vi "Build.vi"(6 "Assembly Type":string, 8 "Position":i32, 9 "XYZTheta":dbl[](array[numeric]), 10 "Pattern Coordinates":dbl[][](array[numeric]), 11 "Dispense in":refnum<class "Dispense.lvclass">) -> (3 "Dispense out":refnum<class "Dispense.lvclass">)   [LabVIEW 2021, in "Dispense.lvclass"]
uses:
  Dispense.lvclass
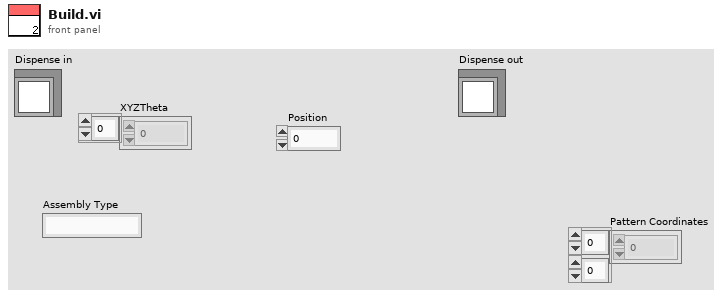
[diagram p1: front panel]
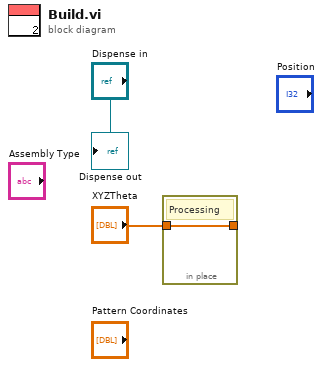
[diagram p0: block diagram]
diagram:
  n1 = in-place "In Place Element Structure" {
    in-place-border: [w3] -> _
    in-place-border: "XYZTheta" -> [w3]
    # "Processing"
  }
  "Dispense out" <- "Dispense in"
